vi "ToggleBool.vi"(11 "Boolean":bool) -> (3 "toggled bool":bool)   [LabVIEW 2019]
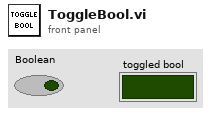
[diagram p1: front panel]
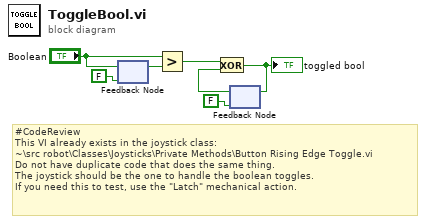
[diagram p0: block diagram]
diagram:
  # "#CodeReview\nThis VI already exists in the joystick class: \n~\\src robot\\Classes\\Joysticks\\Private Methods\\Button Rising Edge Toggle.vi\nDo not have duplicate code that does the same thing.\nThe joystick should be the one to handle the boolean toggles.\nIf you need this to test, use the \"Latch\" mechanical action."
  n1 = feedback #1(FALSE ("Boolean")) -> (w7:bool)
  n2 = feedback-in #1("Boolean") -> ()
  n3 = Greater?(x="Boolean", y=w7) -> (0:w3:bool)
  n4 = feedback #2(FALSE) -> (w2:bool)
  n5 = Exclusive Or(1:w2, 2:w3) -> (0:w1:bool)
  "toggled bool" <- w1
  n6 = feedback-in #2(w1) -> ()
